vi "Data Readers and Writers NEW.vi"(5 "Calling VI Ref":refnum<vi>, 8 "error in (no error)":errorcluster, 9 "(Un)Bundler":refnum<vi>, 10 "Full Element Name":string[](array[string]), 11 "JKI SM in":refnum<class "JKI SM.lvclass">) -> (0 "error out":errorcluster)   [LabVIEW 2013]
uses:
  JKI State Machine API/source/JKI SM/JKI SM.lvclass
  JKI State Machine API/source/JKI SM/JKI SM.lvclass/JKI SM.ctl
  <userlib>/_OpenG.lib/error/error.llb/Filter Error Codes (Array)__ogtk.vi
  <vilib>/regexp/Match Regular Expression.xnode
  <userlib>/_OpenG.lib/comparison/comparison.llb/I32 Changed__ogtk.vi
  <userlib>/_OpenG.lib/comparison/comparison.llb/Boolean Changed__ogtk.vi
panel:
  in  "Listbox":i32(listbox)
  in  "OK":bool
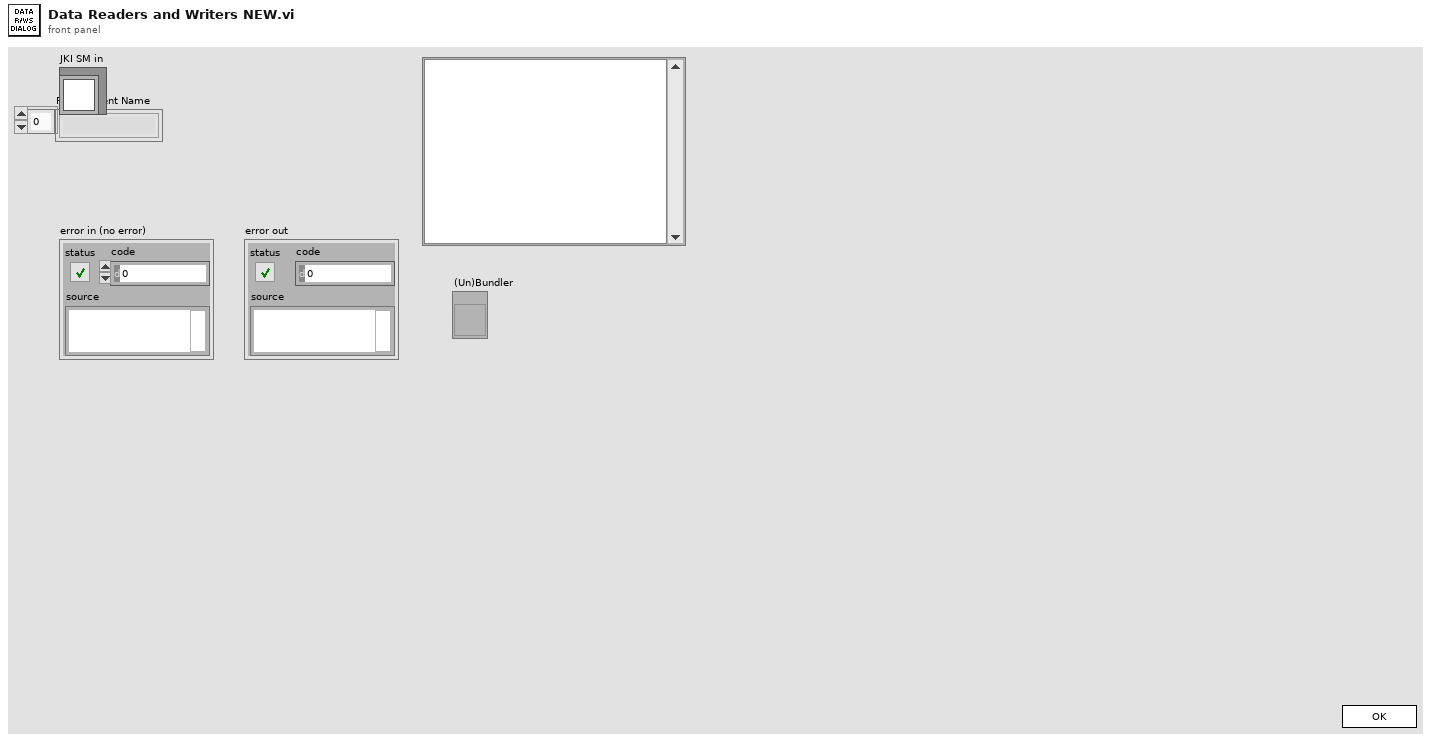
[diagram p1: front panel]
types:
  T1 = enum32{"Invalid", "Standard", "Closed", "Hidden", "Minimized", "Maximized"}
  T2 = enum32{"invalid app kind", "Development System", "Run Time System", "Student Edition", "Embedded LabVIEW", "Evaluation", "Custom"}
  T3 = enum32{"Invalid", "Default", "Floating", "Floating/Auto-Hide", "Modal"}
  T4 = cluster{"Core":cluster{"Current VI Reference":refnum<vi>, "Close Panel on Exit?":bool}, "Your Boolean data":bool, "Your string data":string, "Full Element Name":string[], "JKI SM in":refnum<class "JKI SM.lvclass">, "Callers":cluster{"(Un)Bundler":refnum<vi>, "Structure":string, "Frame Name":string}[], "(Un)Bundler":refnum<vi>}
  T5 = cluster{"(Un)Bundler":refnum<vi>, "Structure":string, "Frame Name":string}[]
  T6 = cluster{"(Un)Bundler":refnum<vi>, "Structure":string, "Frame Name":string}
  T7 = typedef "LVPoint32TypeDef.ctl" = cluster{"Horizontal":i32, "Vertical":i32}
  T8 = cluster{"Shift":bool, "Ctrl":bool, "Alt":bool, "Cmd":bool, "Opt":bool}
  T9 = cluster{"StringConstant":refnum<vi>, "Structure":string, "Frame Name":string}[]
  T10 = cluster{"Current VI Reference":refnum<vi>, "Close Panel on Exit?":bool}
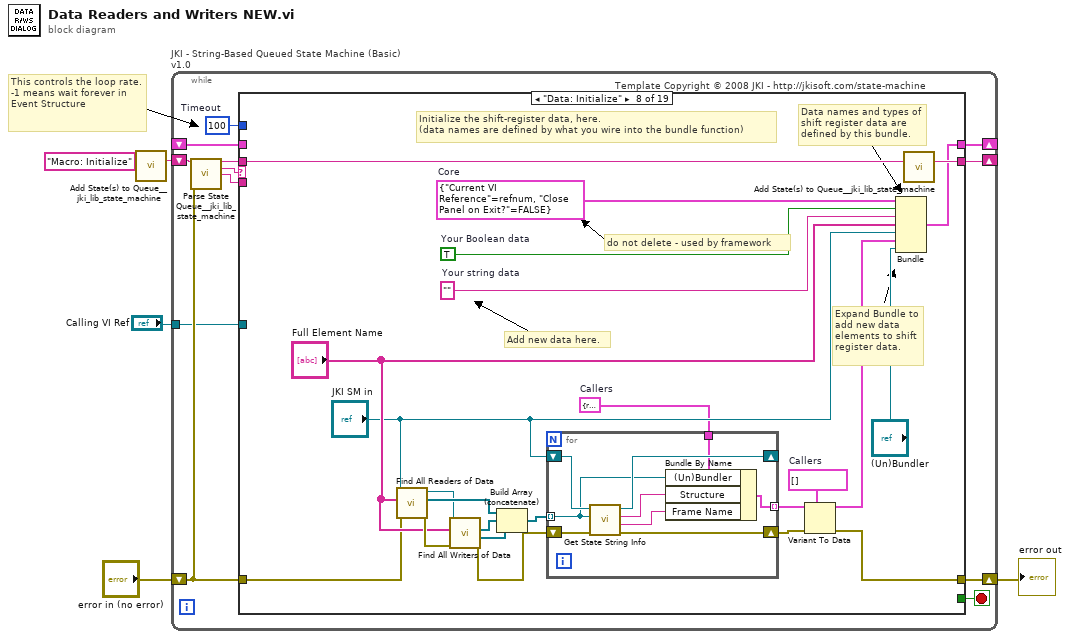
[diagram p0: block diagram]
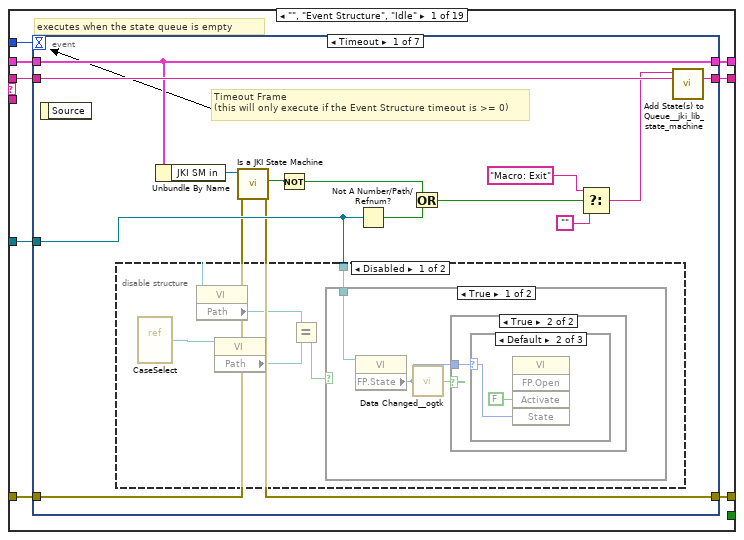
[diagram p2: hidden frame]
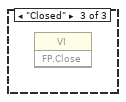
[diagram p5: hidden frame]
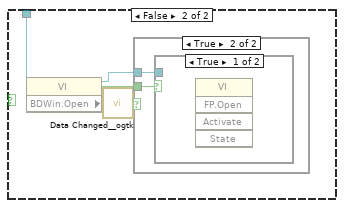
[diagram p6: hidden frame]
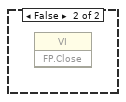
[diagram p8: hidden frame]
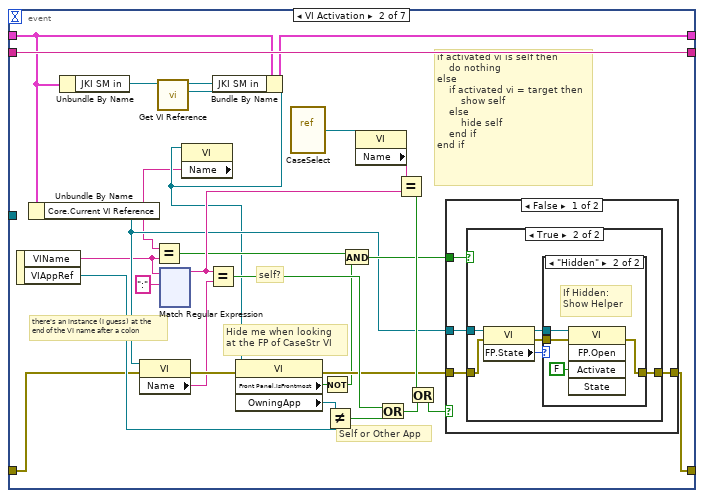
[diagram p10: hidden frame]
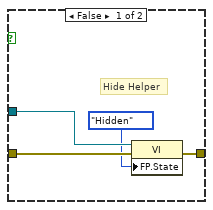
[diagram p11: hidden frame]
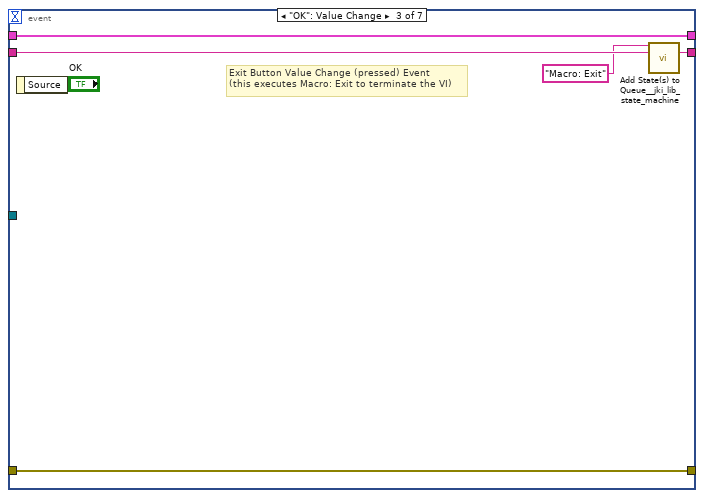
[diagram p14: hidden frame]
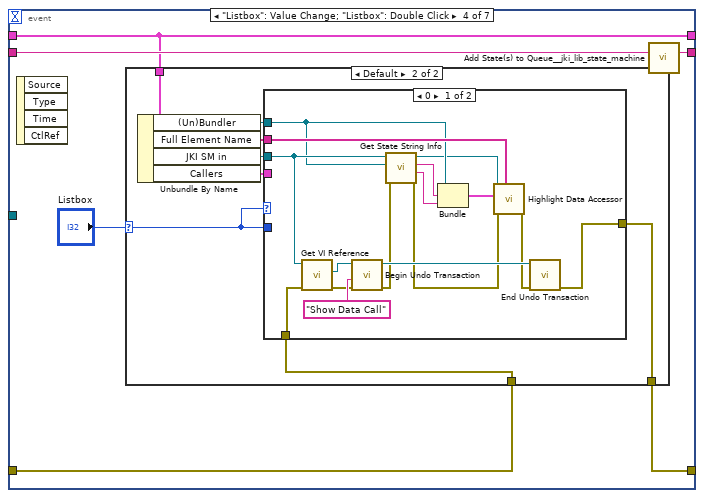
[diagram p15: hidden frame]
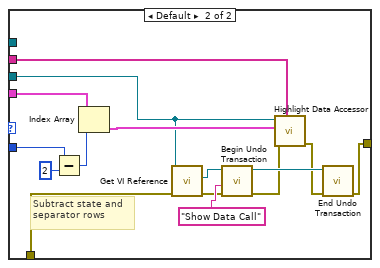
[diagram p17: hidden frame]
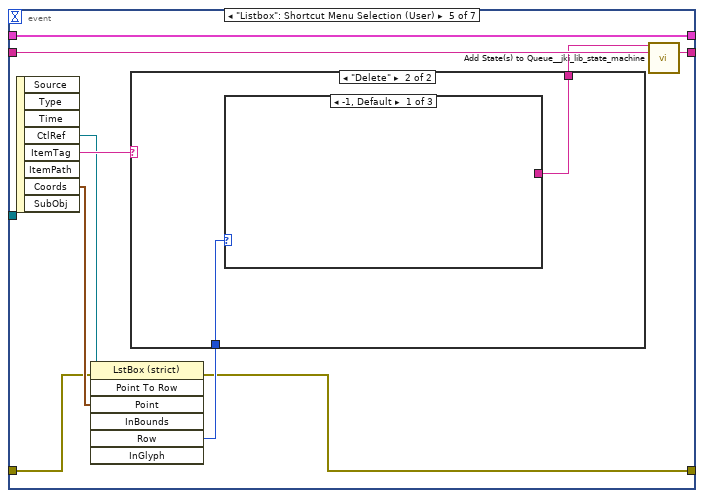
[diagram p18: hidden frame]
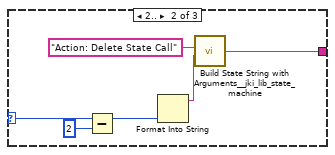
[diagram p20: hidden frame]
diagram:
  # "This controls the loop rate. -1 means wait forever in Event Structure"
  n1 = call <vilib>:"Add State(s) to Queue__jki_lib_state_machine.vi"("State(s) in (\"\")"="Macro: Initialize") -> ("States Out"=w5:string)  [unwired: 14 in]
  n2 = while "JKI - String-Based Queued State Machine (Basic) v1.0" {
    shift-right: [w10] -> _
    shift-left: _ -> [w9]
    shift-right: [w13] -> w3
    shift-left: "error in (no error)" -> [w7]
    shift-right: [w12] -> _
    shift-left: w5 -> [w14]
    tunnel: "Calling VI Ref" -> [w6]
    stop <- w11 stop-if-true
    w8 = 100  # Timeout
    # "Template Copyright © 2008 JKI - http://jkisoft.com/state-machine"
    n3 = call <vilib>:"Parse State Queue__jki_lib_state_machine.vi"("State Queue"=w14, "Error In (no error)"=w7) -> ("Remaining States"=w16:string, "Current State"=w17:string, "Arguments"=w15:string)  [unwired: 11 in]
    n4 = case shown="\"Data: Initialize\"" w17 {
      selector: w17 -> [_ _ w376 _ _ _ _ _ _ _ _ _ _ _ _ _ _ _ _]
      tunnel: w16 -> [w25 w375 w380 w400 w411 w416 w420 w443 w463 w469 w490 w508 w528 w539 w568 w573 w583 w587 w604]
      tunnel: w15 -> [_ _ _ _ _ _ _ _ _ _ _ _ w523 w533 _ _ _ _ _]
      tunnel: w9 -> [w23 w372 w378 w392 w408 w414 w417 _ w460 w466 w488 w502 w526 w535 w565 w571 w580 w584 w600]
      tunnel: [w22 w373 w382 w387 errorcluster {"status"=FALSE, "code"=0, "source"=""} ("error out") w413 w418 w423 w456 w467 w470 w499 w524 w536 w566 w569 w581 w585 w592] -> w13
      tunnel: w7 -> [w21 w373 w381 w388 w406 w413 w418 w432 w454 w467 w470 w500 w525 w537 w566 w569 w581 w585 w601]
      tunnel: [w24 w374 w379 w399 w410 w415 w419 w442 w462 w468 w489 w507 w527 w538 w567 w572 w582 w586 w603] -> w12
      tunnel: [_ _ _ _ _ TRUE _ _ _ _ _ _ _ _ _ _ _ _ _] -> w11
      tunnel: [w20 w372 w378 w398 w408 w414 w417 w441 w460 w466 w488 w502 w526 w535 w565 w571 w580 w584 w589] -> w10
      tunnel: w8 -> [w19 _ _ _ _ _ _ _ _ _ _ _ _ _ _ _ _ _ _]
      tunnel: w6 -> [w18 _ _ _ _ _ _ _ _ _ _ _ _ _ _ _ _ _ _]
      frame "", "Event Structure", "Idle" {
        # "executes when the state queue is empty"
        n5 = event shown="[0] Timeout" {
          selector: _ -> [_ _ _ _ _ _ _]
          dyn-events: _ -> [_ _ _ _ _ _ _]
          timeout: w19 -> [_ _ _ _ _ _ _]
          tunnel: w25 -> [w39 w85 w221 w227 w277 w297 w371]
          tunnel: [w38 w85 w220 w226 w276 w296 w370] -> w24
          tunnel: w23 -> [w33 w59 w218 w225 w269 w295 w368]
          tunnel: [w28 w60 w219 w223 w268 w290 w369] -> w22
          tunnel: w21 -> [w29 w61 w219 w224 w271 w291 w369]
          tunnel: [w33 w58 w218 w225 w269 w295 w368] -> w20
          tunnel: w18 -> [w34 _ _ _ _ _ _]
          event Timeout {
            # "Timeout Frame\n(this will only execute if the Event Structure timeout is >= 0)"
            n6 = event-data() -> ()  [unwired: 1 in, 1 out]
            n7 = disable-structure shown="Disabled" {
              disable-tunnel: w34 -> [w40 _]
              frame Disabled {
                n8 = vi-ref "CaseSelect.vi"() -> (w42:refnum<vi>)
                n9 = property class="VI"(reference=w40) -> ("Path"=w41:path)  [unwired: 1 in, 2 out]
                n10 = property class="VI"(reference=w42) -> ("Path"=w44:path)  [unwired: 1 in, 2 out]
                n11 = Equal?(x=w41, y=w44) -> (x = y?=w43:bool)
                n12 = case shown="True" w43 {
                  tunnel: w40 -> [w45 w52]
                  frame True {
                    n13 = property class="VI"(reference=w45) -> ("FP.State"=w46:T1)  [unwired: 1 in, 2 out]
                    n14 = call-poly <userlib>:"Data Changed__ogtk.vi"("I32"=w46) -> ("Changed"=w47:bool)
                    n15 = case shown="True" w47 {
                      tunnel: w46 -> [_ w48]
                      frame False {
                      }
                      frame True {
                        n16 = case shown="Default" w48 {
                          selector: w48 -> [_ w49 _]
                          frame "Invalid" {
                          }
                          frame Default {
                            n17 = invoke class="VI" method="FP.Open"("Activate"=FALSE ("Activate?"), "State"=w49) -> ()  [unwired: 3 in, 5 out]
                          }
                          frame "Closed" {
                            n18 = invoke class="VI" method="FP.Close"() -> ()  [unwired: 3 in, 3 out]
                          }
                        }
                      }
                    }
                  }
                  frame False {
                    n19 = property class="VI"(reference=w52) -> (reference out=w51:refnum<vi>, "BDWin.Open"=w53:bool)  [unwired: 1 in, 1 out]
                    n20 = call-poly <userlib>:"Data Changed__ogtk.vi"("Boolean"=w53) -> ("Changed"=w54:bool)
                    n21 = case shown="True" w54 {
                      tunnel: w53 -> [_ w56]
                      tunnel: w51 -> [_ w55]
                      frame False {
                      }
                      frame True {
                        n22 = case shown="True" w56 {
                          tunnel: w55 -> [_ _]
                          frame True {
                            n23 = invoke class="VI" method="FP.Open"() -> ()  [unwired: 5 in, 5 out]
                          }
                          frame False {
                            n24 = invoke class="VI" method="FP.Close"() -> ()  [unwired: 3 in, 3 out]
                          }
                        }
                      }
                    }
                  }
                }
              }
              frame Enabled {
              }
            }
            n25 = Unbundle By Name(w33) -> ("JKI SM in"=w32:refnum<class "JKI SM.lvclass">)
            n26 = call "Is a JKI State Machine.vi"("error in (no error)"=w29, "JKI SM in"=w32) -> ("error out"=w28:errorcluster, "Is a JKI State Machine"=w31:bool)  [unwired: 7 in, 1 out]
            n27 = Not(x=w31) -> (.not. x?=w30:bool)
            n28 = Not A Number/Path/Refnum?(number/path/refnum=w34) -> (NaN/Path/Refnum?=w27:bool)
            n29 = Or(x=w30, y=w27) -> (x .or. y?=w26:bool)
            n30 = Select(t="Macro: Exit", s=w26, f="") -> (s? t:f=w35:string)
            n31 = call <vilib>:"Add State(s) to Queue__jki_lib_state_machine.vi"("State(s) in Front (\"\")"=w35, "State(s) in (\"\")"=w39) -> ("States Out"=w38:string)  [unwired: 13 in]
          }
          event VI Activation {
            # "Self or Other App"
            # "self?"
            # "Hide me when looking\nat the FP of CaseStr VI"
            # "there's an instance (I guess) at the\nend of the VI name after a colon"
            # "if activated vi is self then\n    do nothing\nelse\n    if activated vi = target then\n        show self\n    else\n        hide self\n    end if\nend if"
            n32 = event-data() -> ("VIName"=w63:string, "VIAppRef"=w62:refnum<vi>)  [unwired: 1 in]
            n33 = Unbundle By Name(w59) -> ("Core.Current VI Reference"=w70:refnum<vi>)
            n34 = Unbundle By Name(w59) -> ("JKI SM in"=w66:refnum<class "JKI SM.lvclass">)
            n35 = property class="VI"(reference=w70, error in=w61) -> (error out=w74:errorcluster, "Name"=w69:string)  [unwired: 1 out]
            n36 = call "Get VI Reference.vi"("JKI SM in"=w66) -> ("VI"=w65:refnum<vi>, "JKI SM out"=w57:refnum<class "JKI SM.lvclass">)  [unwired: 8 in, 1 out]
            n37 = xnode "Match Regular Expression"("input string"=w63, "regular expression"=":") -> ("before match"=w81:string)  [unwired: 3 in, 5 out]
            n38 = property class="VI"(reference=w65) -> ("Name"=w64:string)  [unwired: 1 in, 2 out]
            n39 = Equal?(x=w64, y=w63) -> (x = y?=w67:bool)
            n40 = Equal?(x=w81, y=w69) -> (x = y?=w78:bool)
            n41 = Bundle By Name(cluster=w59, "JKI SM in"=w57) -> (w58:T4)
            n42 = property class="VI"(reference=w65, error in=w74) -> (error out=w73:errorcluster, "Front Panel.IsFrontmost"=w71:bool, "OwningApp"=w76:refnum<vi>)  [unwired: 1 out]
            n43 = vi-ref "CaseSelect.vi"() -> (w79:refnum<vi>)
            n44 = Not(x=w71) -> (.not. x?=w72:bool)
            n45 = Not Equal?(x=w76, y=w62) -> (x != y?=w77:bool)
            n46 = And(x=w67, y=w72) -> (x .and. y?=w75:bool)
            n47 = property class="VI"(reference=w79) -> ("Name"=w80:string)  [unwired: 1 in, 2 out]
            n48 = Or(x=w78, y=w77) -> (x .or. y?=w83:bool)
            n49 = Equal?(x=w80, y=w81) -> (x = y?=w82:bool)
            n50 = Or(x=w82, y=w83) -> (x .or. y?=w84:bool)
            n51 = case shown="False" w84 {
              tunnel: w73 -> [w89 w105]
              tunnel: [w87 w105] -> w60
              tunnel: w70 -> [w88 _]
              tunnel: w75 -> [w86 _]
              frame False {
                n52 = case shown="True" w86 {
                  tunnel: w89 -> [w93 w98]
                  tunnel: w88 -> [w92 w99]
                  tunnel: [w91 w96] -> w87
                  frame False {
                    # "Hide Helper"
                    n53 = property class="VI"(reference=w92, error in=w93, "FP.State"=T1."Hidden" ("Front Panel Window:State")) -> (error out=w91:errorcluster)  [unwired: 1 out]
                  }
                  frame True {
                    n54 = property class="VI"(reference=w99, error in=w98) -> (reference out=w95:refnum<vi>, error out=w94:errorcluster, "FP.State"=w97:T1)
                    n55 = case shown="\"Hidden\"" w97 {
                      tunnel: [w100 w104] -> w96
                      tunnel: w95 -> [_ w103]
                      tunnel: w94 -> [w100 w102]
                      frame Default {
                      }
                      frame "Hidden" {
                        # "If Hidden:\nShow Helper"
                        n56 = invoke class="VI" method="FP.Open"(reference=w103, error in=w102, "Activate"=FALSE ("Activate?")) -> (error out=w104:errorcluster)  [unwired: 2 in, 4 out]
                      }
                    }
                  }
                }
              }
              frame True {
              }
            }
          }
          event "OK": Value Change {
            # "Exit Button Value Change (pressed) Event\n(this executes Macro: Exit to terminate the VI)"
            n57 = event-data() -> ()  [unwired: 1 in, 1 out]
            n58 = call <vilib>:"Add State(s) to Queue__jki_lib_state_machine.vi"("State(s) in Front (\"\")"="Macro: Exit", "State(s) in (\"\")"=w221) -> ("States Out"=w220:string)  [unwired: 13 in]
          }
          event "Listbox": Value Change; "Listbox": Double Click {
            n59 = event-data() -> ()  [unwired: 1 in, 4 out]
            n60 = case shown="Default" "Listbox" {
              selector: "Listbox" -> [_ w230]
              tunnel: w225 -> [_ w236]
              tunnel: w224 -> [w228 w233]
              tunnel: [w228 w232] -> w223
              frame -1 {
              }
              frame Default {
                n61 = Unbundle By Name(w236) -> ("(Un)Bundler"=w229:refnum<vi>, "Full Element Name"=w231:string[], "JKI SM in"=w234:refnum<class "JKI SM.lvclass">, "Callers"=w235:T5)
                n62 = case shown="0" w230 {
                  tunnel: w235 -> [_ w267]
                  tunnel: w234 -> [w250 w258]
                  tunnel: w233 -> [w251 w254]
                  tunnel: w230 -> [_ w263]
                  tunnel: [w249 w255] -> w232
                  tunnel: w231 -> [w252 w265]
                  tunnel: w229 -> [w248 _]
                  frame 0 {
                    n63 = call "Get VI Reference.vi"("error in (no error)"=w251, "JKI SM in"=w250) -> ("error out"=w246:errorcluster, "VI"=w245:refnum<vi>)  [unwired: 7 in, 1 out]
                    n64 = call "Begin Undo Transaction.vi"("error in (no error)"=w246, "Action"="Show Data Call", "VI in"=w245) -> ("error out"=w238:errorcluster, "VI out"=w244:refnum<vi>)  [unwired: 7 in]
                    n65 = call "Get State String Info.vi"("error in (no error)"=w238, "GObj Refnum in"=w248, "JKI SM in"=w250) -> ("error out"=w237:errorcluster, "Frame Name"=w241:string, "Structure"=w242:string, "JKI SM out"=w243:refnum<class "JKI SM.lvclass">)  [unwired: 5 in]
                    n66 = Bundle("(Un)Bundler"=w248, "Structure"=w242, "Frame Name"=w241) -> (w240:T6)  [unwired: 1 in]
                    n67 = call "Highlight Data Accessor.vi"("Full Element Name"=w252, "error in (no error)"=w237, "Cluster"=w240, "JKI SM in"=w243) -> ("error out"=w239:errorcluster)  [unwired: 6 in, 1 out]
                    n68 = call "End Undo Transaction.vi"("error in (no error)"=w239, "VI in"=w244) -> ("error out"=w249:errorcluster)  [unwired: 8 in, 1 out]
                  }
                  frame Default {
                    # "Subtract state and separator rows"
                    n69 = Subtract(x=w263, y=2) -> (x-y=w262:i32)
                    n70 = Index Array(array=w267, index=w262) -> (element=w266:T6)
                    n71 = call "Get VI Reference.vi"("error in (no error)"=w254, "JKI SM in"=w258) -> ("error out"=w260:errorcluster, "VI"=w259:refnum<vi>)  [unwired: 7 in, 1 out]
                    n72 = call "Begin Undo Transaction.vi"("error in (no error)"=w260, "Action"="Show Data Call", "VI in"=w259) -> ("error out"=w253:errorcluster, "VI out"=w257:refnum<vi>)  [unwired: 7 in]
                    n73 = call "Highlight Data Accessor.vi"("Full Element Name"=w265, "error in (no error)"=w253, "Cluster"=w266, "JKI SM in"=w258) -> ("error out"=w256:errorcluster)  [unwired: 6 in, 1 out]
                    n74 = call "End Undo Transaction.vi"("error in (no error)"=w256, "VI in"=w257) -> ("error out"=w255:errorcluster)  [unwired: 8 in, 1 out]
                  }
                }
              }
            }
            n75 = call <vilib>:"Add State(s) to Queue__jki_lib_state_machine.vi"("State(s) in (\"\")"=w227) -> ("States Out"=w226:string)  [unwired: 14 in]
          }
          event "Listbox": Shortcut Menu Selection (User) {
            n76 = event-data() -> ("CtlRef"=w274:refnum<vi>, "ItemTag"=w275:string, "Coords"=w273:T7)  [unwired: 1 in, 5 out]
            n77 = invoke class="LstBox (strict)" method="Point To Row"(reference=w274, error in=w271, "Point"=w273) -> (error out=w268:errorcluster, "Row"=w272:i32)  [unwired: 4 in, 5 out]
            n78 = case shown="\"Delete\"" w275 {
              tunnel: w272 -> [_ w279]
              tunnel: [_ w278] -> w270
              frame Default {
              }
              frame "Delete" {
                n79 = case shown="-1, Default" w279 {
                  selector: w279 -> [_ w282 _]
                  tunnel: [_ w283 w286] -> w278
                  frame -1, Default {
                  }
                  frame 2.. {
                    n80 = Subtract(x=w282, y=2) -> (x-y=w281:i32)
                    n81 = Format Into String(w281) -> (resulting string=w284:string)  [unwired: 3 in, 1 out]
                    n82 = call <vilib>:"Build State String with Arguments__jki_lib_state_machine.vi"("Arguments (\"\")"=w284, "State"="Action: Delete State Call") -> ("State with Arguments"=w283:string)  [unwired: 4 in]
                  }
                  frame 0 {
                    n83 = call <vilib>:"Build State String with Arguments__jki_lib_state_machine.vi"("State"="Action: Delete State") -> ("State with Arguments"=w286:string)  [unwired: 5 in]
                  }
                }
              }
            }
            n84 = call <vilib>:"Add State(s) to Queue__jki_lib_state_machine.vi"("State(s) in Front (\"\")"=w270, "State(s) in (\"\")"=w277) -> ("States Out"=w276:string)  [unwired: 13 in]
          }
          event Key Down? {
            n85 = event-data() -> ("Char"=w294:i16, "ScanCode"=w289:i16, "PlatMods"=w293:T8)  [unwired: 1 in, 7 out]
            n86 = case shown="Default" w289 {
              tunnel: w295 -> [_ w315]
              tunnel: w294 -> [_ w313]
              tunnel: w293 -> [_ w310]
              tunnel: [_ w308] -> w292
              tunnel: w291 -> [w299 w306]
              tunnel: [w299 w305] -> w290
              tunnel: [w298 _] -> w288
              frame 83 {
                n87 = local read "Listbox"() -> (w300:i32)
                n88 = case shown="Default" w300 {
                  selector: w300 -> [_ w301]
                  tunnel: [_ w302] -> w298
                  frame -1 {
                  }
                  frame Default {
                    n89 = Format Into String(w301) -> (resulting string=w303:string)  [unwired: 3 in, 1 out]
                    n90 = call <vilib>:"Build State String with Arguments__jki_lib_state_machine.vi"("Arguments (\"\")"=w303, "State"="Action: Delete State Call") -> ("State with Arguments"=w302:string)  [unwired: 4 in]
                  }
                }
              }
              frame Default {
                n91 = Unbundle By Name(w315) -> ("JKI SM in"=w307:refnum<class "JKI SM.lvclass">, "Callers"=w314:T5)
                n92 = Build Array(w313) -> (w312:i16[])
                n93 = Unbundle By Name(w310) -> ("Ctrl"=w309:bool)
                n94 = Byte Array To String(unsigned byte array=w312) -> (string=w311:string)
                n95 = case shown="True" w309 {
                  tunnel: w314 -> [_ w324]
                  tunnel: w311 -> [_ w323]
                  tunnel: w310 -> [_ w322]
                  tunnel: [_ w321] -> w308
                  tunnel: w307 -> [_ w319]
                  tunnel: [w316 w318] -> w305
                  tunnel: w306 -> [w316 w317]
                  frame False {
                  }
                  frame True {
                    n96 = To Upper Case(1:w323) -> (0:w320:string)
                    n97 = case shown="\"F\"" w320 {
                      tunnel: w324 -> [_ w339 w349 _]
                      tunnel: w322 -> [_ w334 _ w358]
                      tunnel: [_ TRUE TRUE TRUE] -> w321
                      tunnel: w319 -> [_ _ w342 w355]
                      tunnel: [w325 w332 w340 w352] -> w318
                      tunnel: w317 -> [w325 w332 w341 w356]
                      frame Default {
                      }
                      frame "G" {
                        w327 = 2 ("y")
                        n98 = local read "Listbox"() -> (w329:i32)
                        n99 = Unbundle By Name(w334) -> ("Shift"=w335:bool)
                        n100 = Array Size(array=w339) -> (size(s)=w326:i32)
                        n101 = Subtract(x=w329, y=w327) -> (x-y=w328:i32)
                        n102 = Decrement(x=w328) -> (x-1=w337:i32)
                        n103 = Increment(x=w328) -> (x+1=w338:i32)
                        n104 = Select(t=w337, s=w335, f=w338) -> (s? t:f=w336:i32)
                        n105 = Quotient & Remainder(x=w336, y=w326) -> (x-y*floor(x/y)=w331:i32)  [unwired: 1 out]
                        n106 = Add(x=w331, y=w327) -> (x+y=w330:i32)
                        n107 = property on="Listbox" class="LstBox (strict)"("Val(Sgnl)"=w330) -> ()  [unwired: 2 in, 2 out]
                      }
                      frame "F" {
                        n108 = local read "Listbox"() -> (w350:i32)
                        n109 = Index Array(array=w349, index=w350) -> (element=w348:T6)
                        n110 = Unbundle By Name(w348) -> ("Frame Name"=w344:string)
                        n111 = control-ref of="This VI"() -> (w343:refnum<vi>)
                        n112 = call "Find All Callers of State.vi"("error in (no error)"=w341, "State Name"=w344, "JKI SM in"=w342) -> ("error out"=w345:errorcluster, "Callers"=w346:T9, "JKI SM out"=w347:refnum<class "JKI SM.lvclass">)  [unwired: 6 in]
                        n113 = call "Open Search Results Dialog.vi"("VI Refnum"=w343, "error in (no error)"=w345, "Callers"=w346, "State"=w344, "JKI SM in"=w347) -> ("error out"=w340:errorcluster)  [unwired: 6 in]
                      }
                      frame "Z" {
                        # "Override Ctrl+Z and Ctrl+Shift+Z\n(Handle them here and target the user's VI)"
                        n114 = call "Get VI Reference.vi"("error in (no error)"=w356, "JKI SM in"=w355) -> ("error out"=w353:errorcluster, "VI"=w354:refnum<vi>)  [unwired: 7 in, 1 out]
                        n115 = Unbundle By Name(w358) -> ("Shift"=w357:bool)
                        n116 = case shown="False" w357 {
                          tunnel: w354 -> [w362 w365]
                          tunnel: w353 -> [w360 w364]
                          tunnel: [w361 w363] -> w352
                          frame False {
                            n117 = invoke class="VI" method="Transaction.Undo"(reference=w362, error in=w360) -> (error out=w361:errorcluster)  [unwired: 1 in, 2 out]
                          }
                          frame True {
                            n118 = invoke class="VI" method="Transaction.Redo"(reference=w365, error in=w364) -> (error out=w363:errorcluster)  [unwired: 1 in, 2 out]
                          }
                        }
                      }
                    }
                  }
                }
              }
            }
            n119 = event-data("Discard?"=w292) -> ()  [unwired: 1 in, 1 out]
            n120 = call <vilib>:"Add State(s) to Queue__jki_lib_state_machine.vi"("State(s) in Front (\"\")"=w288, "State(s) in (\"\")"=w297) -> ("States Out"=w296:string)  [unwired: 13 in]
          }
          event Panel Close? {
            # "Discard the event because we'll close the front panel ourselves in Macro: Exit"
            # "Close Panel button (pressed) Event\n(this executes Macro: Exit to terminate the VI)"
            n121 = event-data() -> ()  [unwired: 1 in, 1 out]
            n122 = event-data("Discard?"=TRUE) -> ()  [unwired: 1 in, 1 out]
            n123 = call <vilib>:"Add State(s) to Queue__jki_lib_state_machine.vi"("State(s) in Front (\"\")"="Macro: Exit", "State(s) in (\"\")"=w371) -> ("States Out"=w370:string)  [unwired: 13 in]
          }
        }
      }
      frame "---------- Core ----------" {
        # "Do not put any code in this frame.\n(it is a separator no-op)"
        n124 = call <vilib>:"Add State(s) to Queue__jki_lib_state_machine.vi"("State(s) in (\"\")"=w375) -> ("States Out"=w374:string)  [unwired: 14 in]
      }
      frame Default {
        w385 = 42 items=["No error", "Argument error", "Memory is full", "Out of zone", "End of file", "File already open", "Generic file I/O error", "File not found", "File permission error", "Disk is full", "Duplicate path", "Too many files open", "System feature not enabled", "Resource file not found", "Cannot add resource", "Resource not found", "Image not found", "Image memory error", "Pen does not exist", "Config type invalid", "Config token not found", "Config parse error", "Config memory error", "Bad external code format", "Bad external code offset", "External code not present", "Null window", "Destroy window error", "Null menu", "Print aborted", "Bad print record", "Print driver error", "Windows error during printing", "Memory error during printing", "Print dialog error", "Generic print error", "Invalid device refnum", "Device not found", "Device parameter error", "Device unit error", "Cannot open device", "Device call aborted", "Generic error", "Cancelled by user", "Object ID too low", "Object ID too high", "Object not in heap", "Unknown heap", "Unknown object (invalid DefProc)", "Unknown object (DefProc not in table)", "Message out of range", "Invalid (null) method", "Unknown message", "Manager call not supported", "Bad address", "Network operation in progress", "Network operation timed out", "Connection is busy", "Network attribute not supported", "Network error", "Address in use", "System out of memory", "Connection aborted", "Connection refused", "Not connected", "Already connected", "Connection closed", "Initialization error (interapplication manager)", "Bad occurrence", "Wait on unbound occurrence handler", "Occurrence queue overflow", "Datalog type conflict", "Unused", "Unrecognized type (interapplication manager)", "Memory corrupt", "Failed to make temporary DLL", "Old CIN version", "Drag socket not found", "Failed to load drop-object", "Failed to register OLE object", "Failed to release OLE object", "Format specifier type mismatch", "Unknown format specifier", "Too few format specifiers", "Too many format specifiers", "Scan failed", "Newer CIN version", "Error converting to variant", "Runtime menu error", "Password tampered", "Variant attribute not found", "Incompatible variant data type", "Event data is not available", "Event Store is not present", "Occurrence is not found", "Event Queue is not created", "Event info is not available", "Refnum passed is NULL", "Error retrieving Class GUID", "Error retrieving CoClass GUID", "Error retrieving TypeLib GUID.", "Bad built application magic bytes.", "Specific driver is different from the specific driver associated with the Logical Name.", "There is no session opened to the class driver.", "Max Error", "MAX - Error with config objects", "MAX - Error loading configuration", "MAX - Group not supported"]
        # "Current State"
        # "Do not delete, rename, or modify this frame.\n(this is used to capture unhandled states and typos)"
        # "Handle mistyped state name (developer tool)"
        n125 = Format Into String(format string="Software Exception: Unhandled State \"%s\"." ("message"), error in=w381, w376) -> (resulting string=w384:string, error out=w383:errorcluster)  [unwired: 1 in]
        n126 = call <vilib>:"Error Cluster From Error Code.vi"("show call chain? (False)"=TRUE, "error in (no error)"=w383, "error message (\"\")"=w384, "error code (0)"=w385) -> ("error out"=w382:errorcluster)  [unwired: 5 in]
        n127 = call <vilib>:"Add State(s) to Queue__jki_lib_state_machine.vi"("State(s) in (\"\")"=w380) -> ("States Out"=w379:string)  [unwired: 14 in]
      }
      frame "Initialize Core Data" {
        # "Do not delete, rename, or modify this frame.\n(this is used to determine panel behavior on exit)"
        # "originally closed?"
        # "exe?"
        # "If panel starts closed or is an EXE, then close it when we exit"
        n128 = property class="VI"() -> ("Clone Name"=w390:string)  [unwired: 2 in, 2 out]
        n129 = Open VI Reference(vi path=w390, error in (no error)=w388) -> (vi reference=w389:refnum<vi>, error out=w387:errorcluster)  [unwired: 4 in]
        n130 = property class="VI"() -> ("Front Panel.Open"=w397:bool)  [unwired: 2 in, 2 out]
        n131 = property class="App"() -> ("App.Kind"=w396:T2)  [unwired: 2 in, 2 out]
        n132 = Not(x=w397) -> (.not. x?=w394:bool)
        n133 = Equal?(x=w396, y=T2."Run Time System" ("Application:Kind")) -> (x = y?=w393:bool)
        n134 = Or(x=w394, y=w393) -> (x .or. y?=w391:bool)
        n135 = Bundle By Name(cluster=w392, "Core.Current VI Reference"=w389, "Core.Close Panel on Exit?"=w391) -> (w398:T4)
        n136 = call <vilib>:"Add State(s) to Queue__jki_lib_state_machine.vi"("State(s) in (\"\")"=w400) -> ("States Out"=w399:string)  [unwired: 14 in]
      }
      frame "Error Handler" {
        w407 = i32[] [1026]  # JKI SM VI Invalid Ref
        # "Unhandled Error -- Display it"
        # "Handle any errors here.\nYou can also output any states to clean-up after errors occur"
        # "Clear error"
        n137 = call-poly <userlib>:"Filter Error Codes__ogtk.vi"("Error In"=w406, "Error Codes to Filter"=w407) -> ("Error Out"=w405:errorcluster, "Error Filtered?"=w404:bool)  [unwired: 7 in, 1 out]
        n138 = call <vilib>:"General Error Handler.vi"("error in (no error)"=w405) -> ()  [unwired: 10 in, 5 out]
        n139 = Select(t="Macro: Exit", s=w404, f="") -> (s? t:f=w401:string)
        n140 = call <vilib>:"Add State(s) to Queue__jki_lib_state_machine.vi"("State(s) in Front (\"\")"=w401, "State(s) in (\"\")"=w411) -> ("States Out"=w410:string)  [unwired: 13 in]
      }
      frame "Exit" {
        # "Do not put any code in this frame.\n(No errors that occur here will be handled.)"
        n141 = call <vilib>:"Add State(s) to Queue__jki_lib_state_machine.vi"("State(s) in (\"\")"=w416) -> ("States Out"=w415:string)  [unwired: 14 in]
      }
      frame "---------- Data ----------" {
        # "Do not put any code in this frame.\n(It is a separator no-op. You can make a copy of this frame to create a new Data frame)"
        n142 = call <vilib>:"Add State(s) to Queue__jki_lib_state_machine.vi"("State(s) in (\"\")"=w420) -> ("States Out"=w419:string)  [unwired: 14 in]
      }
      frame "Data: Initialize" {
        w426 = T5 []  # Callers
        w428 = T6 {"(Un)Bundler"=refnum, "Structure"="", "Frame Name"=""}  # Callers
        w438 = T10 {"Current VI Reference"=refnum, "Close Panel on Exit?"=FALSE}  # Core
        w440 = TRUE  # Your Boolean data
        w439 = ""  # Your string data
        # "do not delete - used by framework"
        # "Expand Bundle to add new data elements to shift register data."
        # "Add new data here."
        # "Data names and types of shift register data are defined by this bundle."
        # "Initialize the shift-register data, here.\n(data names are defined by what you wire into the bundle function)"
        n143 = call "Find All Readers of Data.vi"("error in (no error)"=w432, "Full Element Name"="Full Element Name", "JKI SM in"="JKI SM in") -> ("error out"=w435:errorcluster, "NamedUnbundlers"=w437:refnum<vi>[], "JKI SM out"=w434:refnum<class "JKI SM.lvclass">)  [unwired: 6 in]
        n144 = call "Find All Writers of Data.vi"("error in (no error)"=w435, "Full Element Name"="Full Element Name", "JKI SM in"=w434) -> ("error out"=w429:errorcluster, "InPlaceClusterNode"=w421:refnum<vi>[], "NamedBundlers"=w436:refnum<vi>[])  [unwired: 5 in, 1 out]
        n145 = Build Array (concatenate)(w437, w436, w421) -> (w431:refnum<vi>[])
        n146 = for {
          tunnel: w431 -> [w447] mode=indexing
          shift-right: [w451] -> _
          shift-left: "JKI SM in" -> [w452]
          shift-right: [w449] -> w424
          shift-left: w429 -> [w450]
          tunnel: w428 -> [w448]
          tunnel: [w444] -> w427 mode=indexing
          n147 = call "Get State String Info.vi"("error in (no error)"=w450, "GObj Refnum in"=w447, "JKI SM in"=w452) -> ("error out"=w449:errorcluster, "Frame Name"=w445:string, "Structure"=w446:string, "JKI SM out"=w451:refnum<class "JKI SM.lvclass">)  [unwired: 5 in]
          n148 = Bundle By Name(cluster=w448, "(Un)Bundler"=w447, "Structure"=w446, "Frame Name"=w445) -> (w444:T6)
        }
        n149 = Variant To Data(error in=w424, type=w426, Variant=w427) -> (data=w425:T5, error out=w423:errorcluster)
        n150 = Bundle("Core"=w438, "Your Boolean data"=w440, "Your string data"=w439, "Full Element Name"="Full Element Name", "JKI SM in"="JKI SM in", "Callers"=w425, "(Un)Bundler"="(Un)Bundler") -> (w441:T4)  [unwired: 1 in]
        n151 = call <vilib>:"Add State(s) to Queue__jki_lib_state_machine.vi"("State(s) in (\"\")"=w443) -> ("States Out"=w442:string)  [unwired: 14 in]
      }
      frame "Data: Cleanup" {
        # "Ignore Errors\n(e.g. reference already invalid)"
        # "Cleanup any data and references, here.\n(this is called automatically, by the Macro: Exit)"
        n152 = Unbundle By Name(w460) -> ("Core.Current VI Reference"=w461:refnum<vi>, "Callers"=w459:T5)
        n153 = for {
          tunnel: w459 -> [w465] mode=indexing
          tunnel: [w464] -> w458 mode=indexing
          n154 = Unbundle By Name(w465) -> ("(Un)Bundler"=w464:refnum<vi>)
        }
        n155 = Close Reference(reference=w461, error in (no error)=w454) -> (error out=w457:errorcluster)
        n156 = Close Reference(reference=w458, error in (no error)=w454) -> (error out=w455:errorcluster)
        n157 = call <userlib>:"Clear All Errors__ogtk.vi"("Upsteam Error (optional)"=w454, "Error In"=w455) -> ("Error Out"=w453:errorcluster)  [unwired: 2 in]
        n158 = Merge Errors(w457, w453) -> (w456:errorcluster)
        n159 = call <vilib>:"Add State(s) to Queue__jki_lib_state_machine.vi"("State(s) in (\"\")"=w463) -> ("States Out"=w462:string)  [unwired: 14 in]
      }
      frame "---------- UI ----------" {
        # "Do not put any code in this frame.\n(It is a separator no-op. You can make a copy of this frame to create a new UI frame)"
        n160 = call <vilib>:"Add State(s) to Queue__jki_lib_state_machine.vi"("State(s) in (\"\")"=w469) -> ("States Out"=w468:string)  [unwired: 14 in]
      }
      frame "UI: Initialize" {
        # "Initialize the User Interface, here.\n(this is called automatically, by the Macro: Init)"
        n161 = Unbundle By Name(w488) -> ("Core.Current VI Reference"=w487:refnum<vi>, "Full Element Name"=w475:string[], "Callers"=w471:T5)
        n162 = for {
          tunnel: w471 -> [w498] mode=indexing
          tunnel: [w493] -> w481 mode=indexing if=w492
          tunnel: [w493] -> w472 mode=indexing if=w491
          n163 = Unbundle By Name(w498) -> ("Structure"=w494:string, "Frame Name"=w497:string)
          n164 = Equal?(x="EventStructure" ("Structure"), y=w494) -> (x = y?=w492:bool)
          n165 = Format Into String(format string="%s: %s", w494, w497) -> (resulting string=w493:string)  [unwired: 2 in, 1 out]
          n166 = Not(x=w492) -> (.not. x?=w491:bool)
        }
        n167 = call <userlib>:"1D Array to String__ogtk.vi"("delimiter (Tab)"=".", "Array of Strings"=w475) -> ("delimited string"=w473:string)  [unwired: 9 in]
        n168 = Format Into String(format string="Accessors of %s", w473) -> (resulting string=w485:string)  [unwired: 2 in, 1 out]
        n169 = property class="VI"(reference=w487, "Front Panel.Title"=w485) -> ()  [unwired: 1 in, 2 out]
        n170 = Build Array (concatenate)(w473, "" ("format string"), w481, w472) -> (w482:string[])
        n171 = property on="Listbox" class="LstBox (strict)"("Item Names"=w482, "Value"=-1 ("Listbox")) -> (error out=w480:errorcluster, "Item Symbols"=w479:i32[])  [unwired: 2 in, 1 out]
        n172 = Replace Array Subset(array=w479, new element=-1 ("new element/subarray"), index=1) -> (w478:i32[])
        n173 = property on="Listbox" class="LstBox (strict)"(error in=w480, "Item Symbols"=w478) -> ()  [unwired: 1 in, 2 out]
        n174 = call <vilib>:"Add State(s) to Queue__jki_lib_state_machine.vi"("State(s) in (\"\")"=w490) -> ("States Out"=w489:string)  [unwired: 14 in]
      }
      frame "UI: Pre-Test for 0 or 1 Items" {
        n175 = Unbundle By Name(w502) -> ("JKI SM in"=w503:refnum<class "JKI SM.lvclass">, "Full Element Name"=w505:string[], "Callers"=w504:T5)
        n176 = Array Size(array=w504) -> (size(s)=w506:i32)
        n177 = case shown="1" w506 {
          tunnel: w505 -> [_ w512 w516]
          tunnel: [_ "Macro: Exit" "Macro: Exit"] -> w501
          tunnel: w504 -> [_ _ w521]
          tunnel: w503 -> [_ _ w520]
          tunnel: w500 -> [w509 w510 w518]
          tunnel: [w509 w510 w517] -> w499
          frame Default {
          }
          frame 0 {
            n178 = disable-structure shown="Disabled" {
              disable-tunnel: w512 -> [w515 _]
              frame Disabled {
                n179 = Format Into String(format string="State %s has no callers.", w515) -> (resulting string=w513:string)  [unwired: 2 in, 1 out]
                n180 = One Button Dialog(message=w513) -> ()  [unwired: 1 in, 1 out]
              }
              frame Enabled {
              }
            }
          }
          frame 1 {
            n181 = Index Array(array=w521) -> (element=w519:T6)  [unwired: 1 in]
            n182 = call "Highlight Data Accessor.vi"("Full Element Name"=w516, "error in (no error)"=w518, "Cluster"=w519, "JKI SM in"=w520) -> ("error out"=w517:errorcluster)  [unwired: 6 in, 1 out]
          }
        }
        n183 = call <vilib>:"Add State(s) to Queue__jki_lib_state_machine.vi"("State(s) in Front (\"\")"=w501, "State(s) in (\"\")"=w508) -> ("States Out"=w507:string)  [unwired: 13 in]
      }
      frame "UI: Cursor Set" {
        # "Argument"
        # "Set and Unset Cursor Busy.\n(Usage: \"UI: Cursor Set >> Busy|Idle\")"
        n184 = case shown="\"Idle\", Default" w523 {
          tunnel: w525 -> [w530 w532]
          tunnel: [w529 w531] -> w524
          frame "Idle", Default {
            n185 = call <vilib>:"Unset Busy.vi"("error in (no error)"=w530) -> ("error out"=w529:errorcluster)  [unwired: 10 in]
          }
          frame "Busy" {
            n186 = call <vilib>:"Set Busy.vi"("error in (no error)"=w532) -> ("error out"=w531:errorcluster)  [unwired: 9 in, 1 out]
          }
        }
        n187 = call <vilib>:"Add State(s) to Queue__jki_lib_state_machine.vi"("State(s) in (\"\")"=w528) -> ("States Out"=w527:string)  [unwired: 14 in]
      }
      frame "UI: Front Panel State" {
        # "Argument"
        # "Set Front Panel Open or Closed\n(Usage: \"UI: Front Panel State >> Open|Close\")"
        n188 = Unbundle By Name(w535) -> ("Core.Current VI Reference"=w534:refnum<vi>)
        n189 = case shown="\"Open\", Default" w533 {
          tunnel: w537 -> [w543 w559]
          tunnel: [w545 w560] -> w536
          tunnel: w534 -> [w544 w557]
          frame "Open", Default {
            n190 = property class="VI"(reference=w544, error in=w543) -> (reference out=w541:refnum<vi>, error out=w542:errorcluster, "Front Panel.Open"=w540:bool)
            n191 = case shown="False" w540 {
              tunnel: [w548 w554] -> w545
              tunnel: w542 -> [w551 w554]
              tunnel: w541 -> [w550 _]
              frame False {
                # "Setting Floatin here, instead of VI Properties allows the VI to accept keyboard input immediately after openning. (setting it in VI Properties was causing a bug where it wouldn't receive keyboard input until clicking on the VI)"
                n192 = invoke class="VI" method="FP.Open"(reference=w550, error in=w551, "Activate"=TRUE, "State"=T1."Standard") -> (reference out=w547:refnum<vi>, error out=w549:errorcluster)  [unwired: 1 in, 3 out]
                n193 = property class="VI"(reference=w547, error in=w549, "FP.Behavior"=T3."Floating" ("Front Panel Window:Behavior")) -> (error out=w548:errorcluster)  [unwired: 1 out]
              }
              frame True {
              }
            }
          }
          frame "Close" {
            n194 = property class="VI"(reference=w557, error in=w559) -> (reference out=w556:refnum<vi>, error out=w558:errorcluster, "Front Panel.Open"=w555:bool)
            n195 = case shown="True" w555 {
              tunnel: [w561 w564] -> w560
              tunnel: w558 -> [w561 w563]
              tunnel: w556 -> [_ w562]
              frame False {
              }
              frame True {
                n196 = invoke class="VI" method="FP.Close"(reference=w562, error in=w563) -> (error out=w564:errorcluster)  [unwired: 1 in, 2 out]
              }
            }
          }
        }
        n197 = call <vilib>:"Add State(s) to Queue__jki_lib_state_machine.vi"("State(s) in (\"\")"=w539) -> ("States Out"=w538:string)  [unwired: 14 in]
      }
      frame "---------- Macro ----------" {
        # "Do not put any code in this frame.\n(It is a separator no-op. You can make a copy of this frame to create a new Macro frame)"
        n198 = call <vilib>:"Add State(s) to Queue__jki_lib_state_machine.vi"("State(s) in (\"\")"=w568) -> ("States Out"=w567:string)  [unwired: 14 in]
      }
      frame "Macro: Initialize" {
        w570 = "Data: Initialize\nInitialize Core Data\nAction: Sort Items\nUI: Pre-Test for 0 or 1 Items\nUI: Initialize\nUI: Front Panel State >> Open"  # Data: Initialize Initialize Core Data Action: Sort Items UI: Pre-Test for 0 or 1 Items UI: Initialize UI: Front Panel State >> Open
        # "Initialization Macro\n(This is called once, when the VI starts)"
        n199 = call <vilib>:"Add State(s) to Queue__jki_lib_state_machine.vi"("State(s) in Front (\"\")"=w570, "State(s) in (\"\")"=w573) -> ("States Out"=w572:string)  [unwired: 13 in]
      }
      frame "Macro: Exit" {
        # "Exit Macro\n(This is called once, when the VI exits)"
        n200 = Unbundle By Name(w580) -> ("Core.Close Panel on Exit?"=w579:bool)
        n201 = Select(t="UI: Front Panel State >> Close", s=w579, f="") -> (s? t:f=w576:string)
        n202 = call <vilib>:"Add State(s) to Queue__jki_lib_state_machine.vi"("State(s) in (\"\")"=w576, "State(s) at Back (\"\")"="Data: Cleanup\nExit") -> ("States Out"=w574:string)  [unwired: 13 in]
        n203 = call <vilib>:"Add State(s) to Queue__jki_lib_state_machine.vi"("State(s) in Front (\"\")"=w574, "State(s) in (\"\")"=w583) -> ("States Out"=w582:string)  [unwired: 13 in]
      }
      frame "---------- Action ----------" {
        # "Template Separator\n(You can make a copy of, or modify, this frame)"
        n204 = call <vilib>:"Add State(s) to Queue__jki_lib_state_machine.vi"("State(s) in (\"\")"=w587) -> ("States Out"=w586:string)  [unwired: 14 in]
      }
      frame "Action: Sort Items" {
        # "Your code here.\n(You can make a copy of, or modify, this frame)"
        n205 = Unbundle By Name(w600) -> ("Callers"=w598:T5, "JKI SM in"=w599:refnum<class "JKI SM.lvclass">)
        n206 = call "List All Case Frame Names.vi"("error in (no error)"=w601, "JKI SM in"=w599) -> ("error out"=w593:errorcluster, "All Case Structure Frame Names"=w602:string[], "JKI SM out"=w597:refnum<class "JKI SM.lvclass">)  [unwired: 7 in]
        n207 = call "Get VI Event Structure Reference.vi"("error in (no error)"=w593, "JKI SM in"=w597) -> ("error out"=w594:errorcluster, "Event Structure ref"=w596:refnum<vi>)  [unwired: 7 in, 1 out]
        n208 = property class="EvntStruct"(reference=w596, error in=w594) -> (error out=w592:errorcluster, "EventSelectors"=w595:string[])  [unwired: 1 out]
        n209 = for {
          tunnel: w598 -> [w607]
          tunnel: [w606] -> w591 mode=concatenating
          tunnel: w595 -> [w605] mode=indexing
          n210 = for {
            tunnel: w607 -> [w609] mode=indexing
            tunnel: w605 -> [w614]
            tunnel: [w609] -> w606 mode=indexing if=w608
            n211 = Unbundle By Name(w609) -> ("Structure"=w613:string, "Frame Name"=w615:string)
            n212 = Equal?(x="EventStructure" ("Structure"), y=w613) -> (x = y?=w611:bool)
            n213 = Equal?(x=w615, y=w614) -> (x = y?=w610:bool)
            n214 = And(x=w611, y=w610) -> (x .and. y?=w608:bool)
          }
        }
        n215 = for {
          tunnel: w602 -> [w617] mode=indexing
          tunnel: w598 -> [w618]
          tunnel: [w616] -> w590 mode=concatenating
          n216 = for {
            tunnel: w618 -> [w620] mode=indexing
            tunnel: w617 -> [w625]
            tunnel: [w620] -> w616 mode=indexing if=w619
            n217 = Unbundle By Name(w620) -> ("Structure"=w624:string, "Frame Name"=w626:string)
            n218 = Equal?(x="CaseStructure" ("Structure"), y=w624) -> (x = y?=w622:bool)
            n219 = Equal?(x=w626, y=w625) -> (x = y?=w621:bool)
            n220 = And(x=w622, y=w621) -> (x .and. y?=w619:bool)
          }
        }
        n221 = Build Array (concatenate)(w591, w590) -> (w588:T5)
        n222 = call <vilib>:"Add State(s) to Queue__jki_lib_state_machine.vi"("State(s) in (\"\")"=w604) -> ("States Out"=w603:string)  [unwired: 14 in]
        n223 = Bundle By Name(cluster=w600, "Callers"=w588) -> (w589:T4)
      }
    }
  }
  "error out" <- w3
